vi "Get AI REF StringsAndValues.vi"(8 "error in (no error)":errorcluster, 11 "Instrument.Lockin in":refnum<class "Instrument.Lockin.lvclass">) -> (0 "error out":errorcluster, 2 "AI REF StringsAndValues":cluster{string, i32}[](array[cluster]), 3 "Instrument.Lockin out":refnum<class "Instrument.Lockin.lvclass">)   [LabVIEW 2016, in "Instrument.Lockin.lvclass"]
uses:
  Instrument.Lockin.lvclass
  Instrument.Lockin.lvclass/Instrument.Lockin.ctl
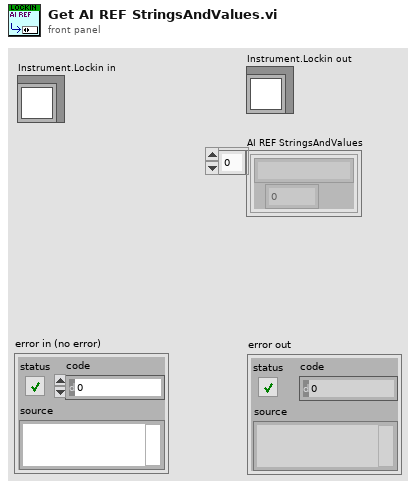
[diagram p1: front panel]
types:
  T1 = typedef "Lockin.DAQ.lvclass/AI.config-array.ctl" = T2[]
  T2 = typedef "Lockin.DAQ.lvclass/AI.config-cluster.ctl" = cluster{"AI.channels":tag, "AI.Coupling":T3, "AI.Range":T4, "input terminal configuration":i32, "DAQ Type":T5}
  T3 = typedef "Lockin.DAQ.lvclass/AI.coupling-enum.ctl" = u16
  T4 = typedef "Lockin.DAQ.lvclass/446xAI-enum.ctl" = enum16{"±0.316 V", "±1.00 V", "±3.16 V", "±10.0 V", "±31.6 V", "±42.4 V"}
  T5 = typedef "Lockin.DAQ.lvclass/DAQType-enum.ctl" = enum16{"None", "USB 4431", "PXI 446x"}
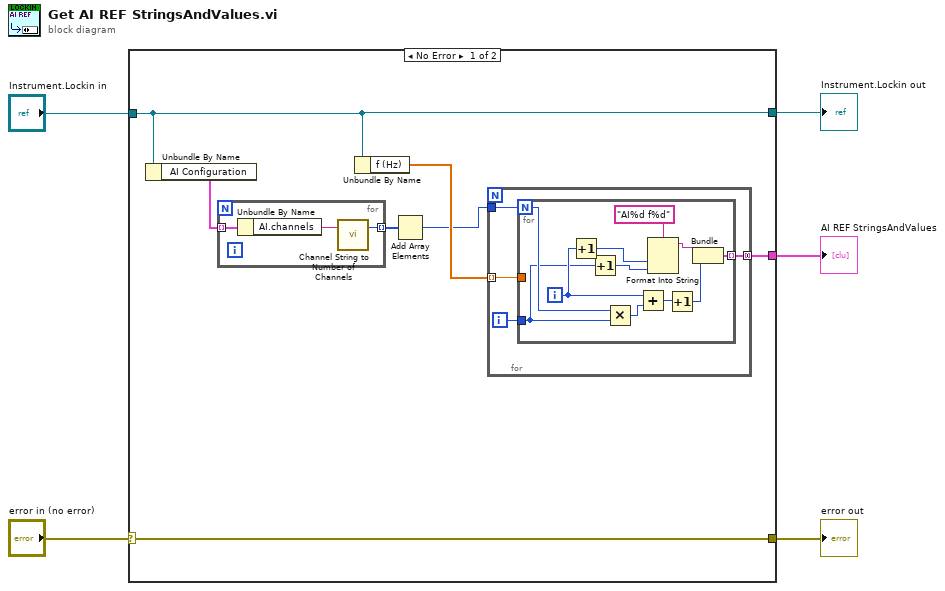
[diagram p0: block diagram]
diagram:
  n1 = case shown="No Error" "error in (no error)" {
    selector: "error in (no error)" -> [w7 w31]
    tunnel: [w10 _] -> w5
    tunnel: "Instrument.Lockin in" -> [w8 w32]
    tunnel: [w8 w32] -> w3
    tunnel: [w7 w31] -> w1
    frame No Error {
      n2 = Unbundle By Name(w8) -> ("AI Configuration"=w12:T1)
      n3 = for {
        tunnel: w12 -> [w15] mode=indexing
        tunnel: [w14] -> w11 mode=indexing
        n4 = Unbundle By Name(w15) -> ("AI.channels"=w13:tag)
        n5 = call "Channel String to Number of Channels.vi"("Channels String"=w13) -> ("# channels"=w14:i32)  [unwired: 2 in]
      }
      n6 = Unbundle By Name(w8) -> ("f (Hz)"=w9:dbl[])
      n7 = Add Array Elements(numeric array=w11) -> (sum=w6:i32)
      n8 = for {
        tunnel: w9 -> [w17] mode=indexing
        tunnel: [w18] -> w10 mode=concatenating
        tunnel: w6 -> [w16]
        i -> [w19]
        n9 = for {
          N: w16 -> [w25]
          tunnel: [w30] -> w18 mode=indexing
          tunnel: w19 -> [w21]
          tunnel: w17 -> [_]
          i -> [w23]
          n10 = Increment(x=w23) -> (x+1=w22:i32)
          n11 = Increment(x=w21) -> (x+1=w20:i32)
          n12 = Multiply(x=w25, y=w21) -> (x*y=w24:i32)
          n13 = Add(x=w23, y=w24) -> (x+y=w29:i32)
          n14 = Format Into String(format string="AI%d f%d", w22, w20) -> (resulting string=w27:string)  [unwired: 2 in, 1 out]
          n15 = Increment(x=w29) -> (x+1=w26:i32)
          n16 = Bundle(w27, w26) -> (w30:cluster{string, i32})  [unwired: 1 in]
        }
      }
    }
    frame Error {
    }
  }
  "AI REF StringsAndValues" <- w5
  "Instrument.Lockin out" <- w3
  "error out" <- w1
